vi "RFmxSpecAn Sample(Harms).vi"(8 "error in (no error)":errorcluster, 10 "# of Harms":u8, 11 "Resource In":refnum<k15> caption="Resource Name") -> (0 "error out":errorcluster, 2 "Harms Results dBm":dbl[][](array[numeric]))   [LabVIEW 2018]
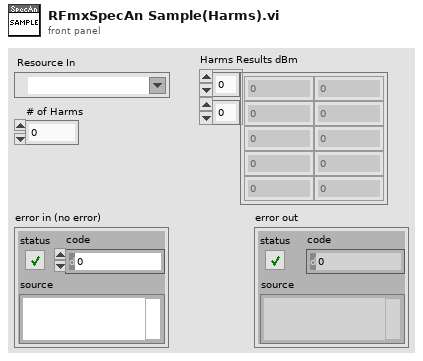
[diagram p1: front panel]
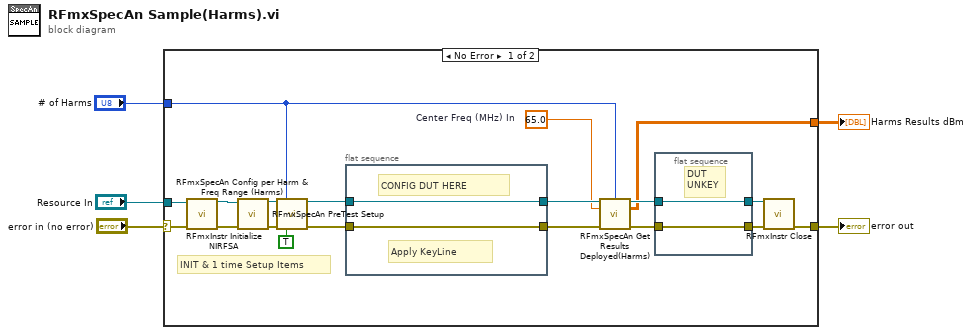
[diagram p0: block diagram]
diagram:
  n1 = case shown="No Error" "error in (no error)" {
    selector: "error in (no error)" -> [w24 w29]
    tunnel: [w11 w29] -> w4
    tunnel: "Resource In" -> [w21 _]
    tunnel: "# of Harms" -> [w13 _]
    tunnel: [w6 _] -> w1
    frame No Error {
      w12 = 65.0  # Center Freq (MHz) In
      # "INIT & 1 time Setup Items"
      n2 = call <vilib>:"RFmxInstr Initialize NIRFSA.vi"("Resource Name"=w21, "error in (no error)"=w24) -> ("Instrument Handle Out"=w22:refnum<k21>, "error out"=w23:errorcluster)  [unwired: 11 in, 1 out]
      n3 = call "RFmxSpecAn PreTest Setup.vi"("error in (no error)"=w23, "Instrument Handle In"=w22) -> ("error out"=w20:errorcluster, "Instrument Handle out"=w19:refnum<k21>)  [unwired: 8 in]
      n4 = call "RFmxSpecAn Config per Harm & Freq Range (Harms).vi"("SA Handle In"=w19, "# of Harms"=w13, "error in (no error)"=w20, "Read Config File"=TRUE) -> ("SA Handle Out"=w15:refnum<k21>, "error out"=w17:errorcluster)  [unwired: 9 in, 1 out]
      n5 = flat-sequence {
        tunnel: w17 -> [w28]
        tunnel: [w28] -> w16
        tunnel: w15 -> [w27]
        tunnel: [w27] -> w14
        frame #0 {
          # "Apply KeyLine"
          # "CONFIG DUT HERE"
        }
      }
      n6 = call "RFmxSpecAn Get Results Deployed(Harms).vi"("SA Handle In"=w14, "# of Harms"=w13, "Center Freq (MHz) In"=w12, "error in (no error)"=w16) -> ("SA Handle Out"=w9:refnum<k21>, "Harms Results dBm"=w6:dbl[][], "error out"=w10:errorcluster)  [unwired: 9 in]
      n7 = flat-sequence {
        tunnel: w10 -> [w25]
        tunnel: w9 -> [w26]
        tunnel: [w26] -> w8
        tunnel: [w25] -> w7
        frame #0 {
          # "DUT\nUNKEY"
        }
      }
      n8 = call <vilib>:"RFmxInstr Close.vi"("Instrument Handle In"=w8, "error in (no error)"=w7) -> ("error out"=w11:errorcluster)  [unwired: 13 in]
    }
    frame Error {
    }
  }
  "error out" <- w4
  "Harms Results dBm" <- w1
